vi "Update Methods Registration.vi"(8 "error in (no error)":errorcluster, 11 "Server class in":refnum<vi>) -> (0 "error out":errorcluster, 3 "Server class out":refnum<vi>)   [LabVIEW 2019, in "gRPC Scripting Tools.lvlib"]
uses:
  gRPC Scripting Tools.lvlib
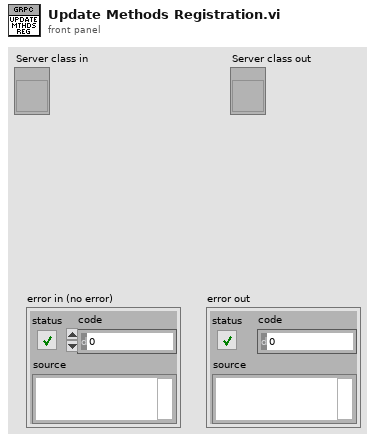
[diagram p1: front panel]
types:
  T1 = typedef "LVPointTypeDef.ctl" = cluster{"Horizontal":i16, "Vertical":i16}
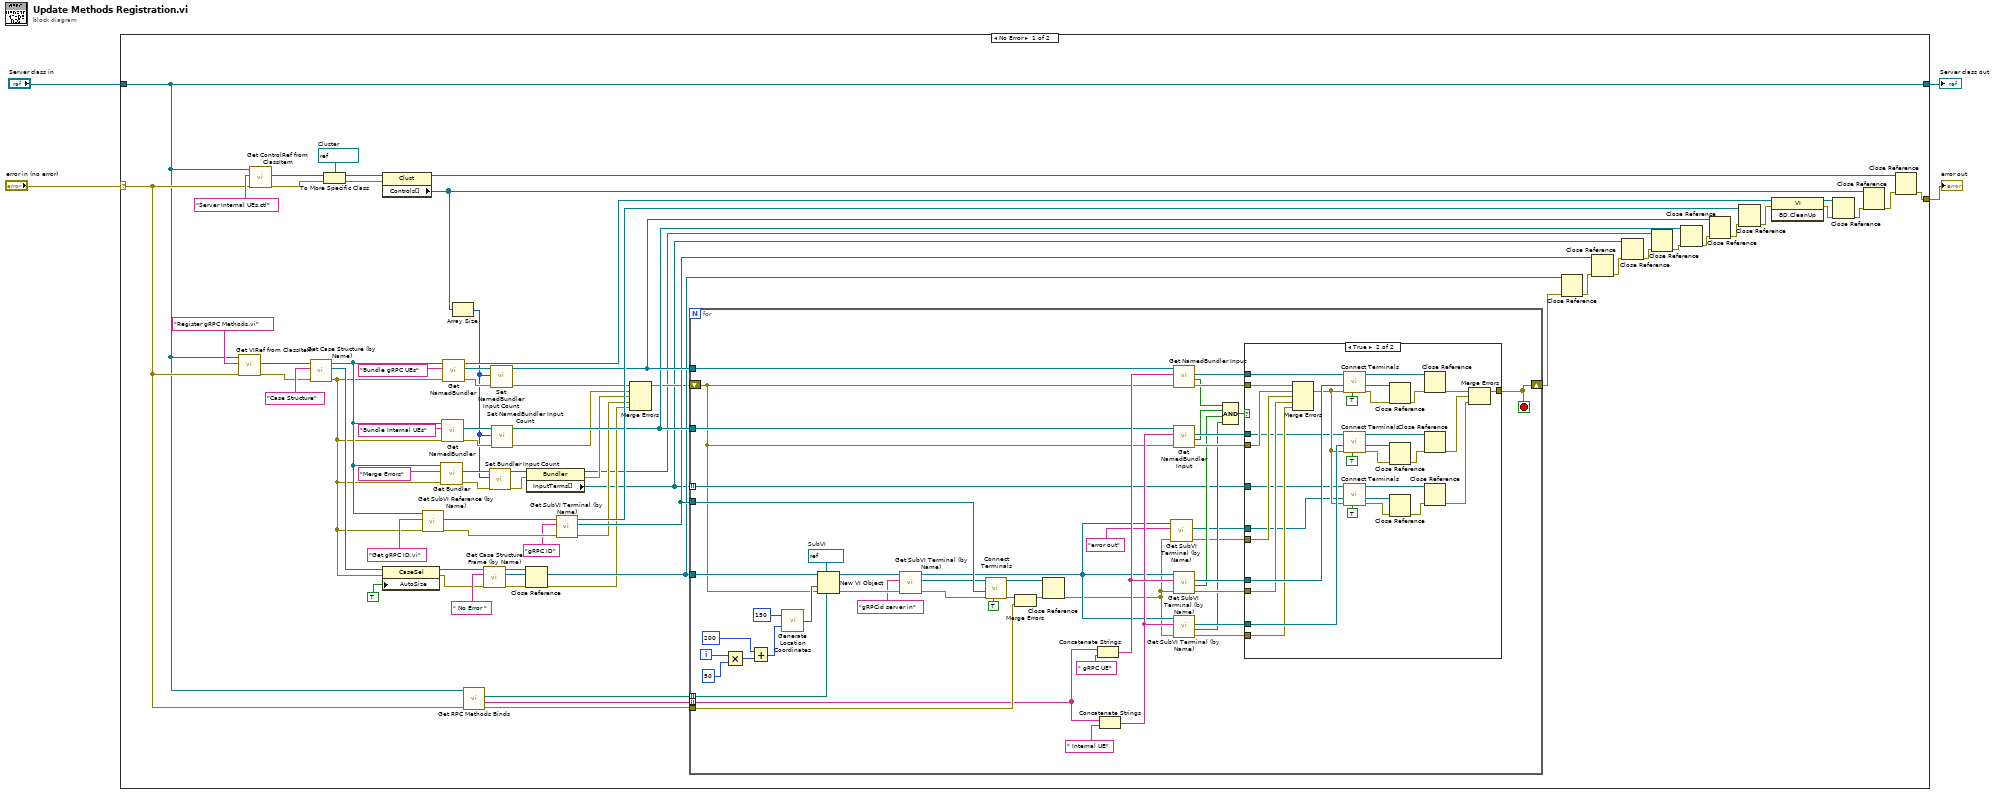
[diagram p0: block diagram]
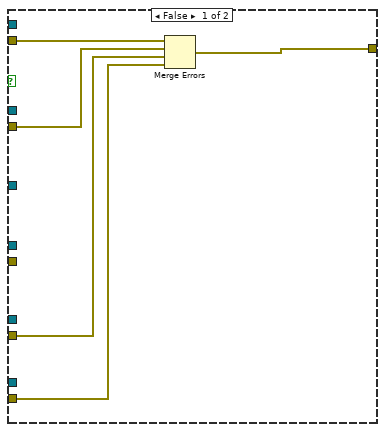
[diagram p2: hidden frame]
diagram:
  n1 = case shown="No Error" "error in (no error)" {
    selector: "error in (no error)" -> [w28 w152]
    tunnel: [w33 w152] -> w4
    tunnel: "Server class in" -> [w27 w153]
    tunnel: [w27 w153] -> w1
    frame No Error {
      w66 = refnum<vi> refnum  # Cluster
      n2 = call "Get VIRef from ClassItem.vi"("error in (no error)"=w28, "Item Name"="Register gRPC Methods.vi", "LVClassLibrary in"=w27) -> ("error out"=w61:errorcluster, "VIref out"=w23:refnum<vi>)  [unwired: 5 in, 2 out]
      n3 = call "Get ControlRef from ClassItem.vi"("error in (no error)"=w28, "Item Name"="Server Internal UEs.ctl", "LVClassLibrary in"=w27) -> ("error out"=w67:errorcluster, "Control ref out"=w65:refnum<vi>)  [unwired: 5 in, 2 out]
      n4 = call "Get Case Structure (by Name).vi"("error in (no error)"=w61, "Case Structure name"="Case Structure" ("y"), "VI ref in"=w23) -> ("error out"=w17:errorcluster, "CaseStructure out"=w39:refnum<vi>, "VI ref out"=w21:refnum<vi>)  [unwired: 5 in, 1 out]
      n5 = To More Specific Class(target class=w66, reference=w65, error in=w67) -> (specific class reference=w68:refnum<vi>, error out=w70:errorcluster)
      n6 = property class="Clust"(reference=w68, error in=w70) -> (reference out=w35:refnum<vi>, "Controls[]"=w69:refnum<vi>[])  [unwired: 1 out]
      n7 = property class="CaseSel"(reference=w39, error in=w17, "AutoSize"=TRUE ("AutoSize To Fit Contents?")) -> (reference out=w38:refnum<vi>, error out=w37:errorcluster)
      n8 = call "Get SubVI Reference (by Name).vi"("error in (no error)"=w17, "SubVI Name"="Get gRPC ID.vi", "Owner VI in"=w21) -> ("error out"=w54:errorcluster, "SubVI Refnum out"=w55:refnum<vi>)  [unwired: 5 in, 2 out]
      n9 = call "Get Bundler.vi"("error in (no error)"=w17, "Label"="Merge Errors", "Owner VI in"=w21) -> ("error out"=w16:errorcluster, "Bundler ref out"=w20:refnum<vi>)  [unwired: 5 in, 2 out]
      n10 = call "Get NamedBundler.vi"("error in (no error)"=w17, "Label"="Bundle Internal UEs" ("name/order"), "Owner VI in"=w21) -> ("error out"=w57:errorcluster, "NamedBundler ref out"=w58:refnum<vi>)  [unwired: 5 in, 2 out]
      n11 = call "Get NamedBundler.vi"("error in (no error)"=w17, "Label"="Bundle gRPC UEs" ("name/order"), "Owner VI in"=w21) -> ("error out"=w59:errorcluster, "NamedBundler ref out"=w72:refnum<vi>, "Owner VI out"=w32:refnum<vi>)  [unwired: 5 in, 1 out]
      n12 = Array Size(array=w69) -> (size(s)=w19:i32)
      n13 = call "Get RPC Methods Binds.vi"("error in (no error)"=w28, "LVClassLibrary in"=w27) -> ("error out"=w26:errorcluster, "RPC Method Binds Names"=w24:string[], "RPC Method Binds Paths"=w25:path[])  [unwired: 6 in, 1 out]
      n14 = call "Get Case Structure Frame (by Name).vi"("error in (no error)"=w37, "element"=" No Error ", "CaseStructure in"=w38) -> ("error out"=w49:errorcluster, "Frame ref out"=w41:refnum<vi>, "CaseStructure out"=w40:refnum<vi>)  [unwired: 5 in, 1 out]
      n15 = call "Set Bundler Input Count.vi"("error in (no error)"=w16, "Numeric"=w19, "Bundler in"=w20) -> ("error out"=w15:errorcluster, "Bundler out"=w18:refnum<vi>)  [unwired: 7 in]
      n16 = call "Set NamedBundler Input Count.vi"("error in (no error)"=w59, "Numeric"=w19, "NamedBundler in"=w72) -> ("error out"=w12:errorcluster, "NamedBundler out"=w51:refnum<vi>)  [unwired: 7 in]
      n17 = call "Set NamedBundler Input Count.vi"("error in (no error)"=w57, "Numeric"=w19, "NamedBundler in"=w58) -> ("error out"=w42:errorcluster, "NamedBundler out"=w50:refnum<vi>)  [unwired: 7 in]
      n18 = Close Reference(reference=w40, error in (no error)=w49) -> (error out=w10:errorcluster)
      n19 = property class="Bundler"(reference=w18, error in=w15) -> (reference out=w6:refnum<vi>, error out=w14:errorcluster, "InputTerms[]"=w8:refnum<vi>[])
      n20 = call "Get SubVI Terminal (by Name).vi"("error in (no error)"=w54, "Terminal name"="gRPC ID", "SubVI in"=w55) -> ("error out"=w13:errorcluster, "SubVI Term ref"=w48:refnum<vi>, "SubVI out"=w52:refnum<vi>)  [unwired: 5 in, 1 out]
      n21 = Merge Errors(w12, w42, w14, w13, w10) -> (w11:errorcluster)
      n22 = for {
        tunnel: w41 -> [w121]
        tunnel: w51 -> [w120]
        tunnel: w50 -> [w112]
        tunnel: w48 -> [w96]
        tunnel: w25 -> [w83] mode=indexing
        tunnel: w26 -> [w82]
        tunnel: w24 -> [w81] mode=indexing
        tunnel: w8 -> [w76] mode=indexing
        shift-right: [w105] -> w47
        shift-left: w11 -> [w74]
        i -> [w94]
        stop <- w105 stop-if-true
        w119 = refnum<vi> refnum  # SubVI
        n23 = Multiply(x=w94, y=50) -> (x*y=w92:i32)
        n24 = Add(x=i16 200 ("Horizontal"), y=w92) -> (x+y=w90:i32)
        n25 = call "Generate Location Coordinates.vi"("Vertical"=w90, "Horizontal"=i16 150) -> ("Location out"=w89:T1)
        n26 = New VI Object(vi object class=w119, owner refnum=w121, position/next to=w89, 6:w83, 8:w74) -> (object refnum=w98:refnum<vi>, 0:w99:errorcluster)  [unwired: 3 in]
        n27 = call "Get SubVI Terminal (by Name).vi"("error in (no error)"=w99, "Terminal name"="gRPCid server in", "SubVI in"=w98) -> ("error out"=w86:errorcluster, "SubVI Term ref"=w87:refnum<vi>, "SubVI out"=w80:refnum<vi>)  [unwired: 5 in, 1 out]
        n28 = call "Connect Terminals.vi"("Auto Route? (F)"=TRUE, "Error In"=w86, "Source Terminal"=w96, "Sink Terminal"=w87) -> ("Error Out"=w85:errorcluster)  [unwired: 7 in]
        n29 = Merge Errors(w85, w82) -> (w84:errorcluster)
        n30 = Close Reference(reference=w87, error in (no error)=w84) -> (error out=w78:errorcluster)
        n31 = Concatenate Strings(w81, " gRPC UE" ("string")) -> (w115:string)
        n32 = Concatenate Strings(w81, " Internal UE" ("string")) -> (w113:string)
        n33 = call "Get SubVI Terminal (by Name).vi"("error in (no error)"=w78, "Terminal name"="error out", "SubVI in"=w80) -> ("error out"=w77:errorcluster, "SubVI Term ref"=w75:refnum<vi>)  [unwired: 5 in, 2 out]
        n34 = call "Get NamedBundler Input.vi"("error in (no error)"=w74, "Input name"=w115, "NamedBundler ref in"=w120) -> ("error out"=w109:errorcluster, "Found?"=w104:bool, "Input Term ref"=w118:refnum<vi>)  [unwired: 5 in, 1 out]
        n35 = call "Get NamedBundler Input.vi"("error in (no error)"=w74, "Input name"=w113, "NamedBundler ref in"=w112) -> ("error out"=w107:errorcluster, "Found?"=w103:bool, "Input Term ref"=w111:refnum<vi>)  [unwired: 5 in, 1 out]
        n36 = call "Get SubVI Terminal (by Name).vi"("error in (no error)"=w78, "Terminal name"=w115, "SubVI in"=w80) -> ("error out"=w108:errorcluster, "Found?"=w102:bool, "SubVI Term ref"=w117:refnum<vi>)  [unwired: 5 in, 1 out]
        n37 = call "Get SubVI Terminal (by Name).vi"("error in (no error)"=w78, "Terminal name"=w113, "SubVI in"=w80) -> ("error out"=w106:errorcluster, "Found?"=w101:bool, "SubVI Term ref"=w110:refnum<vi>)  [unwired: 5 in, 1 out]
        n38 = Compound Arithmetic op=AND(w104, w103, w102, w101) -> (w100:bool)
        n39 = case shown="True" w100 {
          tunnel: w118 -> [_ w130]
          tunnel: w117 -> [_ w148]
          tunnel: w111 -> [_ w133]
          tunnel: w110 -> [_ w147]
          tunnel: w109 -> [w126 w146]
          tunnel: w108 -> [w123 w143]
          tunnel: w107 -> [w124 w145]
          tunnel: w106 -> [w122 w142]
          tunnel: [w125 w151] -> w105
          tunnel: w77 -> [_ w144]
          tunnel: w76 -> [_ w138]
          tunnel: w75 -> [_ w136]
          frame False {
            n40 = Merge Errors(w126, w124, w123, w122) -> (w125:errorcluster)
          }
          frame True {
            n41 = Merge Errors(w146, w145, w144, w143, w142) -> (w140:errorcluster)
            n42 = call "Connect Terminals.vi"("Auto Route? (F)"=TRUE, "Error In"=w140, "Source Terminal"=w148, "Sink Terminal"=w130) -> ("Error Out"=w128:errorcluster)  [unwired: 7 in]
            n43 = call "Connect Terminals.vi"("Auto Route? (F)"=TRUE, "Error In"=w140, "Source Terminal"=w147, "Sink Terminal"=w133) -> ("Error Out"=w134:errorcluster)  [unwired: 7 in]
            n44 = call "Connect Terminals.vi"("Auto Route? (F)"=TRUE, "Error In"=w140, "Source Terminal"=w136, "Sink Terminal"=w138) -> ("Error Out"=w137:errorcluster)  [unwired: 7 in]
            n45 = Close Reference(reference=w148, error in (no error)=w128) -> (error out=w129:errorcluster)
            n46 = Close Reference(reference=w147, error in (no error)=w134) -> (error out=w132:errorcluster)
            n47 = Close Reference(reference=w136, error in (no error)=w137) -> (error out=w139:errorcluster)
            n48 = Close Reference(reference=w130, error in (no error)=w129) -> (error out=w127:errorcluster)
            n49 = Close Reference(reference=w133, error in (no error)=w132) -> (error out=w131:errorcluster)
            n50 = Close Reference(reference=w138, error in (no error)=w139) -> (error out=w135:errorcluster)
            n51 = Merge Errors(w127, w131, w135) -> (w151:errorcluster)
          }
        }
      }
      n52 = Close Reference(reference=w41, error in (no error)=w47) -> (error out=w46:errorcluster)
      n53 = Close Reference(reference=w48, error in (no error)=w46) -> (error out=w9:errorcluster)
      n54 = Close Reference(reference=w8, error in (no error)=w9) -> (error out=w7:errorcluster)
      n55 = Close Reference(reference=w6, error in (no error)=w7) -> (error out=w5:errorcluster)
      n56 = Close Reference(reference=w50, error in (no error)=w5) -> (error out=w45:errorcluster)
      n57 = Close Reference(reference=w51, error in (no error)=w45) -> (error out=w44:errorcluster)
      n58 = Close Reference(reference=w52, error in (no error)=w44) -> (error out=w31:errorcluster)
      n59 = invoke class="VI" method="BD.CleanUp"(reference=w32, error in=w31) -> (reference out=w30:refnum<vi>, error out=w29:errorcluster)  [unwired: 1 in, 1 out]
      n60 = Close Reference(reference=w30, error in (no error)=w29) -> (error out=w43:errorcluster)
      n61 = Close Reference(reference=w69, error in (no error)=w43) -> (error out=w34:errorcluster)
      n62 = Close Reference(reference=w35, error in (no error)=w34) -> (error out=w33:errorcluster)
    }
    frame Error {
    }
  }
  "error out" <- w4
  "Server class out" <- w1
